vi "appendCircStrArr.vi"(7 "Buffer Length":i32, 8 "error in (no error)":errorcluster, 9 "New String":string, 10 "String Array":string[](array[string]), 11 "MatOper in":refnum<class "MatOper.lvclass">) -> (0 "error out":errorcluster, 2 "Updated String Array":string[](array[string]), 3 "MatOper out":refnum<class "MatOper.lvclass">)   [LabVIEW 2016, in "OfcFunc.lvlib" / "MatOper.lvclass"]
doc: "Append the circular string array based on the buffer length."
uses:
  MatOper.lvclass
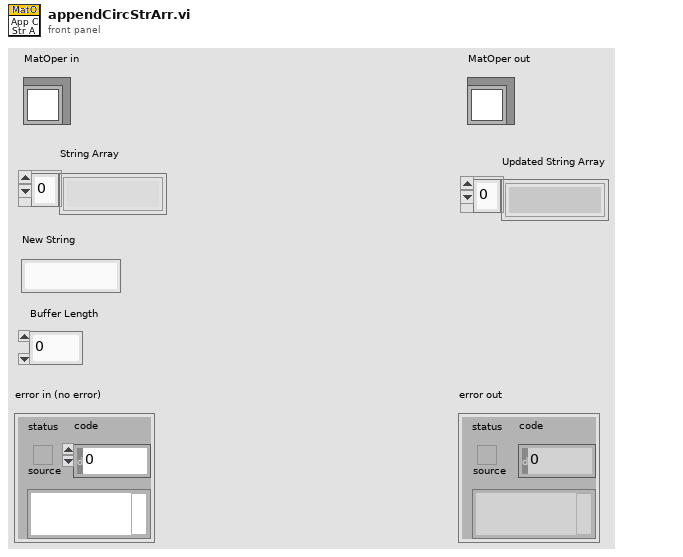
[diagram p1: front panel]
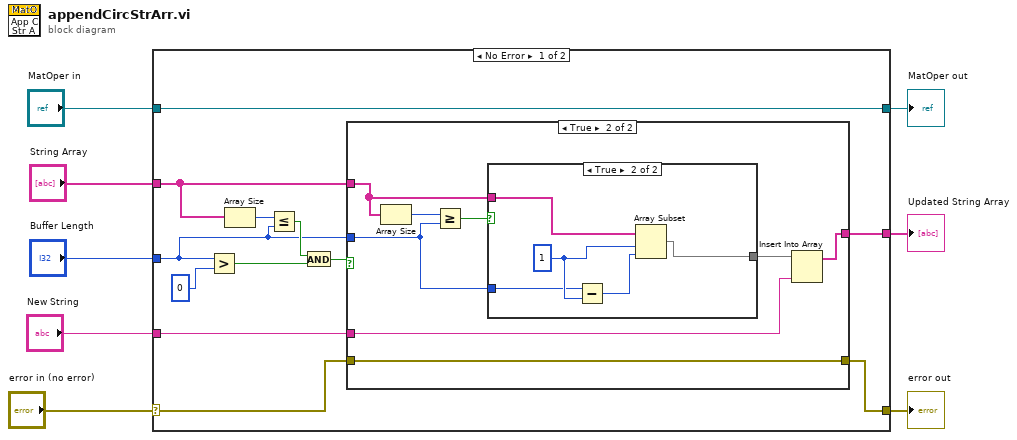
[diagram p0: block diagram]
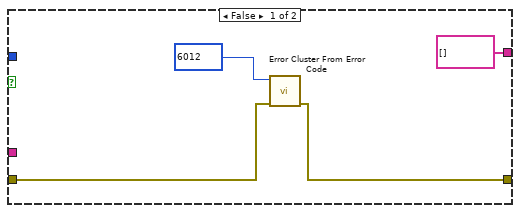
[diagram p2: hidden frame]
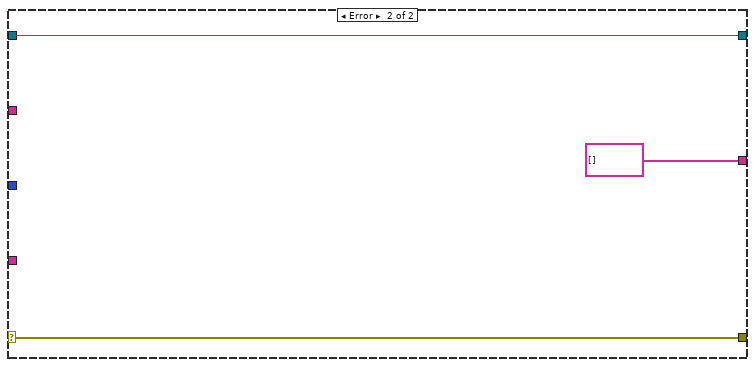
[diagram p4: hidden frame]
diagram:
  n1 = case shown="No Error" "error in (no error)" {
    selector: "error in (no error)" -> [w16 w41]
    tunnel: [w15 w41] -> w7
    tunnel: [w20 w40] -> w5
    tunnel: "MatOper in" -> [w20 w40]
    tunnel: "String Array" -> [w13 _]
    tunnel: "Buffer Length" -> [w9 _]
    tunnel: "New String" -> [w19 _]
    tunnel: [w18 string[] [] ("String Array")] -> w1
    frame No Error {
      n2 = Greater?(x=w9, y=0) -> (0:w10:bool)
      n3 = Array Size(array=w13) -> (size(s)=w14:i32)
      n4 = Less Or Equal?(x=w14, y=w9) -> (x <= y?=w11:bool)
      n5 = And(x=w11, y=w10) -> (x .and. y?=w12:bool)
      n6 = case shown="True" w12 {
        tunnel: w13 -> [_ w30]
        tunnel: w19 -> [_ w26]
        tunnel: [string[] [] ("String Array") w28] -> w18
        tunnel: w9 -> [_ w27]
        tunnel: w16 -> [w22 w25]
        tunnel: [w21 w25] -> w15
        frame False {
          n7 = call <vilib>:"Error Cluster From Error Code.vi"("error in (no error)"=w22, "error code (0)"=6012) -> ("error out"=w21:errorcluster)  [unwired: 7 in]
        }
        frame True {
          n8 = Array Size(array=w30) -> (size(s)=w32:i32)
          n9 = Greater Or Equal?(x=w32, y=w27) -> (x >= y?=w31:bool)
          n10 = case shown="True" w31 {
            tunnel: w30 -> [w33 w38]
            tunnel: [w33 w34] -> w29
            tunnel: w27 -> [_ w36]
            frame False {
            }
            frame True {
              w37 = 1 ("index")
              n11 = Subtract(x=w36, y=w37) -> (x-y=w35:i32)
              n12 = Array Subset(array=w38, index=w37, length=w35) -> (w34:string[])
            }
          }
          n13 = Insert Into Array(array=w29, new element=w26) -> (w28:string[])  [unwired: 1 in]
        }
      }
    }
    frame Error {
    }
  }
  "error out" <- w7
  "MatOper out" <- w5
  "Updated String Array" <- w1
